vi "IDByteToNotes.vi"(1 "ID Byte":i32=138) -> (0 "Notes":string)   [LabVIEW 2010]
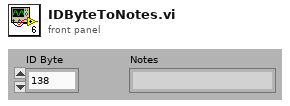
[diagram p1: front panel]
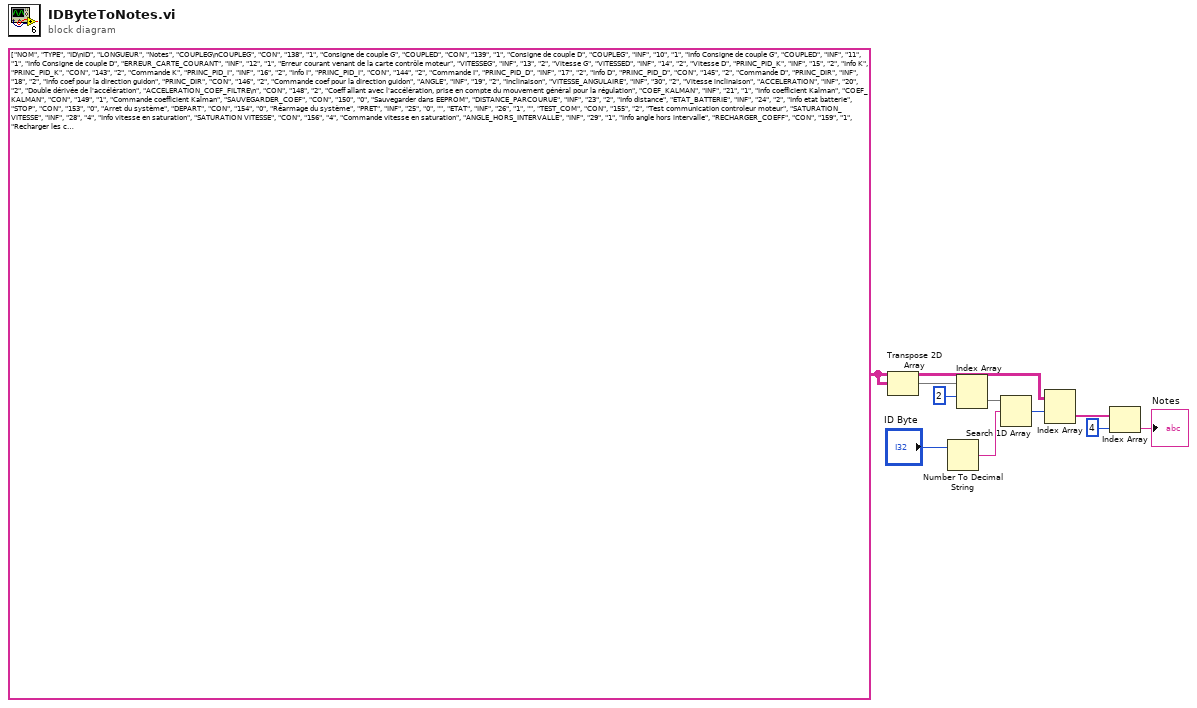
[diagram p0: block diagram]
diagram:
  w6 = string[][] [["NOM", "TYPE", "ID\nID", "LONGUEUR", "Notes"], ["COUPLEG\nCOUPLEG", "CON", "138", "1", "Consigne de couple G"], ["COUPLED", "CON", "139", "1", "Consigne de couple D"], ["COUPLEG", "INF", "10", "1", "Info Consigne de couple G"], ["COUPLED", "INF", "11", "1", "Info Consigne de couple D"], ["ERREUR_CARTE_COURANT", "INF", "12", "1", "Erreur courant venant de la carte contrôle moteur"], ["VITESSEG", "INF", "13", "2", "Vitesse G"], ["VITESSED", "INF", "14", "2", "Vitesse D"], ["PRINC_PID_K", "INF", "15", "2", "Info K"], ["PRINC_PID_K", "CON", "143", "2", "Commande K"], ["PRINC_PID_I", "INF", "16", "2", "Info I"], ["PRINC_PID_I", "CON", "144", "2", "Commande I"], ["PRINC_PID_D", "INF", "17", "2", "Info D"], ["PRINC_PID_D", "CON", "145", "2", "Commande D"], ["PRINC_DIR", "INF", "18", "2", "Info coef pour la direction guidon"], ["PRINC_DIR", "CON", "146", "2", "Commande coef pour la direction guidon"], ["ANGLE", "INF", "19", "2", "Inclinaison"], ["VITESSE_ANGULAIRE", "INF", "30", "2", "Vitesse inclinaison"], ["ACCELERATION", "INF", "20", "2", "Double dérivée de l'accélération"], ["ACCELERATION_COEF_FILTRE\n", "CON", "148", "2", "Coeff allant avec l'accélération, prise en compte du mouvement général pour la régulation"], ["COEF_KALMAN", "INF", "21", "1", "Info coefficient Kalman"], ["COEF_KALMAN", "CON", "149", "1", "Commande coefficient Kalman"], ["SAUVEGARDER_COEF", "CON", "150", "0", "Sauvegarder dans EEPROM"], ["DISTANCE_PARCOURUE", "INF", "23", "2", "Info distance"], ["ETAT_BATTERIE", "INF", "24", "2", "Info etat batterie"], ["STOP", "CON", "153", "0", "Arret du système"], ["DEPART", "CON", "154", "0", "Réarmage du système"], ["PRET", "INF", "25", "0", ""], ["ETAT", "INF", "26", "1", ""], ["TEST_COM", "CON", "155", "2", "Test communication controleur moteur"], ["SATURATION_VITESSE", "INF", "28", "4", "Info vitesse en saturation"], ["SATURATION VITESSE", "CON", "156", "4", "Commande vitesse en saturation"], ["ANGLE_HORS_INTERVALLE", "INF", "29", "1", "Info angle hors intervalle"], ["RECHARGER_COEFF", "CON", "159", "1", "Recharger les coefficients"]]
  n1 = Transpose 2D Array(2D array=w6) -> (transposed array=w4:string[][])
  n2 = Number To Decimal String(number="ID Byte") -> (decimal integer string=w3:string)  [unwired: 1 in]
  n3 = Index Array(array=w4, index (row)=2 ("indice (ligne)")) -> (element=w2:string[])  [unwired: 1 in]
  n4 = Search 1D Array(1D array=w2, element=w3) -> (index of element=w5:i32)  [unwired: 1 in]
  n5 = Index Array(array=w6, index (row)=w5) -> (element=w7:string[])  [unwired: 1 in]
  n6 = Index Array(array=w7, index=4 ("indice")) -> (element=→"Notes":string)
